vi "IDToSubnetAddress.vi"() -> ()   [LabVIEW 2016]
uses:
  ILCID.ctl
panel:
  out "Address":i16
  out "Subnet":i16
  in  "ILCID":T1
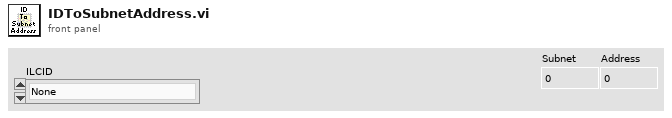
[diagram p1: front panel]
types:
  T1 = typedef "ILCID.ctl" = enum8{"None", "HP1", "HP2", "HP3", "HP4", "HP5", "HP6", "HM1", "HM2", "HM3", "HM4", "HM5", "HM6", "FA101", "FA102", "FA103", "FA104", "FA105", "FA106", "FA107", "FA108", "FA109", "FA110", "FA111", "FA112", "FA113", "FA114", "FA115", "FA116", "FA117", "FA118", "FA119", "FA120", "FA121", "FA122", "FA123", "FA124", "FA125", "FA126", "FA127", "FA128", "FA129", "FA130", "FA131", "FA132", "FA133", "FA134", "FA135", "FA136", "FA137", "FA138", "FA139", "FA140", "FA141", "FA142", "FA143", "FA207", "FA208", "FA209", "FA210", "FA211", "FA212", "FA214", "FA215", "FA216", "FA217", "FA218", "FA219", "FA220", "FA221", "FA222", "FA223", "FA224", "FA225", "FA227", "FA228", "FA229", "FA230", "FA231", "FA232", "FA233", "FA234", "FA235", "FA236", "FA237", "FA238", "FA239", "FA240", "FA241", "FA242", "FA243", "FA301", "FA302", "FA303", "FA304", "FA305", "FA306", "FA307", "FA308", "FA309", "FA310", "FA311", "FA312", "FA313", "FA314", "FA315", "FA316", "FA317", "FA318", "FA319", "FA320", "FA321", "FA322", "FA323", "FA324", "FA325", "FA326", "FA327", "FA328", "FA329", "FA330", "FA331", "FA332", "FA333", "FA334", "FA335", "FA336", "FA337", "FA338", "FA339", "FA340", "FA341", "FA342", "FA343", "FA407", "FA408", "FA409", "FA410", "FA411", "FA412", "FA414", "FA415", "FA416", "FA417", "FA418", "FA419", "FA420", "FA421", "FA422", "FA423", "FA424", "FA425", "FA427", "FA428", "FA429", "FA430", "FA431", "FA432", "FA433", "FA434", "FA435", "FA436", "FA437", "FA438", "FA439", "FA440", "FA441", "FA442", "FA443"}
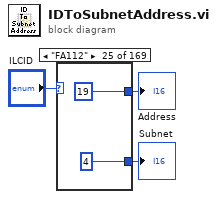
[diagram p0: block diagram]
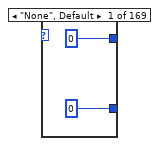
[diagram p2: hidden frame]
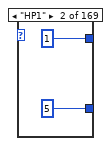
[diagram p3: hidden frame]
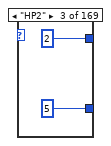
[diagram p4: hidden frame]
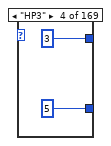
[diagram p5: hidden frame]
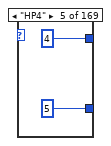
[diagram p6: hidden frame]
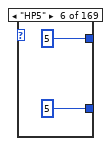
[diagram p7: hidden frame]
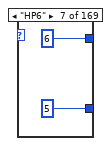
[diagram p8: hidden frame]
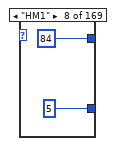
[diagram p9: hidden frame]
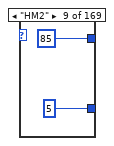
[diagram p10: hidden frame]
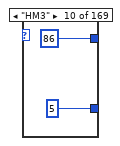
[diagram p11: hidden frame]
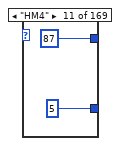
[diagram p12: hidden frame]
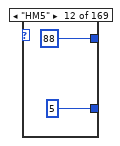
[diagram p13: hidden frame]
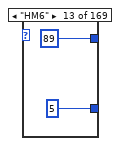
[diagram p14: hidden frame]
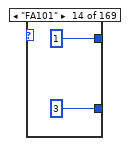
[diagram p15: hidden frame]
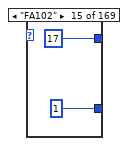
[diagram p16: hidden frame]
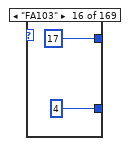
[diagram p17: hidden frame]
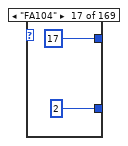
[diagram p18: hidden frame]
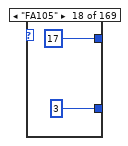
[diagram p19: hidden frame]
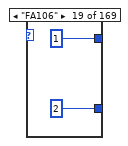
[diagram p20: hidden frame]
diagram:
  n1 = case shown="\"FA112\"" "ILCID" {
    tunnel: [i16 0 i16 5 i16 5 i16 5 i16 5 i16 5 i16 5 i16 5 i16 5 i16 5 i16 5 i16 5 i16 5 i16 3 i16 1 i16 4 i16 2 i16 3 i16 2 i16 1 i16 4 i16 2 i16 3 i16 1 i16 4 i16 2 i16 3 i16 1 i16 4 i16 2 i16 3 i16 2 i16 1 i16 4 i16 2 i16 3 i16 1 i16 4 i16 2 i16 3 i16 1 i16 4 i16 2 i16 3 i16 1 i16 4 i16 2 i16 3 i16 4 i16 2 i16 3 i16 1 i16 4 i16 1 i16 2 i16 3 i16 1 i16 4 i16 2 i16 3 i16 1 i16 4 i16 3 i16 1 i16 4 i16 2 i16 3 i16 2 i16 1 i16 4 i16 2 i16 3 i16 1 i16 4 i16 3 i16 1 i16 4 i16 2 i16 3 i16 1 i16 4 i16 2 i16 3 i16 4 i16 2 i16 3 i16 1 i16 4 i16 1 i16 2 i16 3 i16 3 i16 1 i16 4 i16 2 i16 3 i16 2 i16 1 i16 4 i16 2 i16 3 i16 1 i16 4 i16 2 i16 3 i16 1 i16 4 i16 2 i16 3 i16 2 i16 1 i16 4 i16 2 i16 3 i16 1 i16 4 i16 2 i16 3 i16 1 i16 4 i16 2 i16 3 i16 1 i16 4 i16 2 i16 3 i16 4 i16 2 i16 3 i16 1 i16 4 i16 1 i16 2 i16 3 i16 1 i16 4 i16 2 i16 3 i16 1 i16 4 i16 3 i16 1 i16 4 i16 2 i16 3 i16 2 i16 1 i16 4 i16 2 i16 3 i16 1 i16 4 i16 3 i16 1 i16 4 i16 2 i16 3 i16 1 i16 4 i16 2 i16 3 i16 4 i16 2 i16 3 i16 1 i16 4 i16 1 i16 2 i16 3] -> w2
    tunnel: [i16 0 i16 1 i16 2 i16 3 i16 4 i16 5 i16 6 i16 84 i16 85 i16 86 i16 87 i16 88 i16 89 i16 1 i16 17 i16 17 i16 17 i16 17 i16 1 i16 1 i16 18 i16 18 i16 18 i16 18 i16 19 i16 19 i16 19 i16 19 i16 19 i16 20 i16 20 i16 2 i16 20 i16 21 i16 21 i16 21 i16 21 i16 1 i16 22 i16 22 i16 22 i16 22 i16 23 i16 2 i16 23 i16 23 i16 24 i16 23 i16 2 i16 25 i16 24 i16 2 i16 3 i16 3 i16 3 i16 3 i16 4 i16 24 i16 26 i16 24 i16 24 i16 25 i16 26 i16 25 i16 26 i16 27 i16 27 i16 4 i16 26 i16 27 i16 28 i16 28 i16 27 i16 4 i16 29 i16 28 i16 28 i16 29 i16 4 i16 29 i16 29 i16 30 i16 30 i16 5 i16 31 i16 31 i16 5 i16 6 i16 6 i16 5 i16 5 i16 6 i16 30 i16 30 i16 32 i16 32 i16 6 i16 7 i16 31 i16 33 i16 33 i16 31 i16 32 i16 34 i16 34 i16 32 i16 33 i16 35 i16 35 i16 7 i16 33 i16 34 i16 36 i16 36 i16 34 i16 7 i16 37 i16 37 i16 35 i16 35 i16 38 i16 7 i16 36 i16 36 i16 39 i16 38 i16 8 i16 40 i16 39 i16 8 i16 9 i16 9 i16 8 i16 8 i16 10 i16 37 i16 41 i16 40 i16 37 i16 38 i16 41 i16 38 i16 39 i16 42 i16 42 i16 9 i16 39 i16 40 i16 43 i16 43 i16 40 i16 10 i16 44 i16 41 i16 41 i16 44 i16 9 i16 42 i16 42 i16 45 i16 45 i16 11 i16 26 i16 46 i16 11 i16 12 i16 12 i16 10 i16 10] -> w1
    frame "None", Default {
    }
    frame "HP1" {
    }
    frame "HP2" {
    }
    frame "HP3" {
    }
    frame "HP4" {
    }
    frame "HP5" {
    }
    frame "HP6" {
    }
    frame "HM1" {
    }
    frame "HM2" {
    }
    frame "HM3" {
    }
    frame "HM4" {
    }
    frame "HM5" {
    }
    frame "HM6" {
    }
    frame "FA101" {
    }
    frame "FA102" {
    }
    frame "FA103" {
    }
    frame "FA104" {
    }
    frame "FA105" {
    }
    frame "FA106" {
    }
    frame "FA107" {
    }
    frame "FA108" {
    }
    frame "FA109" {
    }
    frame "FA110" {
    }
    frame "FA111" {
    }
    frame "FA112" {
    }
    frame "FA113" {
    }
    frame "FA114" {
    }
    frame "FA115" {
    }
    frame "FA116" {
    }
    frame "FA117" {
    }
    frame "FA118" {
    }
    frame "FA119" {
    }
    frame "FA120" {
    }
    frame "FA121" {
    }
    frame "FA122" {
    }
    frame "FA123" {
    }
    frame "FA124" {
    }
    frame "FA125" {
    }
    frame "FA126" {
    }
    frame "FA127" {
    }
    frame "FA128" {
    }
    frame "FA129" {
    }
    frame "FA130" {
    }
    frame "FA131" {
    }
    frame "FA132" {
    }
    frame "FA133" {
    }
    frame "FA134" {
    }
    frame "FA135" {
    }
    frame "FA136" {
    }
    frame "FA137" {
    }
    frame "FA138" {
    }
    frame "FA139" {
    }
    frame "FA140" {
    }
    frame "FA141" {
    }
    frame "FA142" {
    }
    frame "FA143" {
    }
    frame "FA207" {
    }
    frame "FA208" {
    }
    frame "FA209" {
    }
    frame "FA210" {
    }
    frame "FA211" {
    }
    frame "FA212" {
    }
    frame "FA214" {
    }
    frame "FA215" {
    }
    frame "FA216" {
    }
    frame "FA217" {
    }
    frame "FA218" {
    }
    frame "FA219" {
    }
    frame "FA220" {
    }
    frame "FA221" {
    }
    frame "FA222" {
    }
    frame "FA223" {
    }
    frame "FA224" {
    }
    frame "FA225" {
    }
    frame "FA227" {
    }
    frame "FA228" {
    }
    frame "FA229" {
    }
    frame "FA230" {
    }
    frame "FA231" {
    }
    frame "FA232" {
    }
    frame "FA233" {
    }
    frame "FA234" {
    }
    frame "FA235" {
    }
    frame "FA236" {
    }
    frame "FA237" {
    }
    frame "FA238" {
    }
    frame "FA239" {
    }
    frame "FA240" {
    }
    frame "FA241" {
    }
    frame "FA242" {
    }
    frame "FA243" {
    }
    frame "FA301" {
    }
    frame "FA302" {
    }
    frame "FA303" {
    }
    frame "FA304" {
    }
    frame "FA305" {
    }
    frame "FA306" {
    }
    frame "FA307" {
    }
    frame "FA308" {
    }
    frame "FA309" {
    }
    frame "FA310" {
    }
    frame "FA311" {
    }
    frame "FA312" {
    }
    frame "FA313" {
    }
    frame "FA314" {
    }
    frame "FA315" {
    }
    frame "FA316" {
    }
    frame "FA317" {
    }
    frame "FA318" {
    }
    frame "FA319" {
    }
    frame "FA320" {
    }
    frame "FA321" {
    }
    frame "FA322" {
    }
    frame "FA323" {
    }
    frame "FA324" {
    }
    frame "FA325" {
    }
    frame "FA326" {
    }
    frame "FA327" {
    }
    frame "FA328" {
    }
    frame "FA329" {
    }
    frame "FA330" {
    }
    frame "FA331" {
    }
    frame "FA332" {
    }
    frame "FA333" {
    }
    frame "FA334" {
    }
    frame "FA335" {
    }
    frame "FA336" {
    }
    frame "FA337" {
    }
    frame "FA338" {
    }
    frame "FA339" {
    }
    frame "FA340" {
    }
    frame "FA341" {
    }
    frame "FA342" {
    }
    frame "FA343" {
    }
    frame "FA407" {
    }
    frame "FA408" {
    }
    frame "FA409" {
    }
    frame "FA410" {
    }
    frame "FA411" {
    }
    frame "FA412" {
    }
    frame "FA414" {
    }
    frame "FA415" {
    }
    frame "FA416" {
    }
    frame "FA417" {
    }
    frame "FA418" {
    }
    frame "FA419" {
    }
    frame "FA420" {
    }
    frame "FA421" {
    }
    frame "FA422" {
    }
    frame "FA423" {
    }
    frame "FA424" {
    }
    frame "FA425" {
    }
    frame "FA427" {
    }
    frame "FA428" {
    }
    frame "FA429" {
    }
    frame "FA430" {
    }
    frame "FA431" {
    }
    frame "FA432" {
    }
    frame "FA433" {
    }
    frame "FA434" {
    }
    frame "FA435" {
    }
    frame "FA436" {
    }
    frame "FA437" {
    }
    frame "FA438" {
    }
    frame "FA439" {
    }
    frame "FA440" {
    }
    frame "FA441" {
    }
    frame "FA442" {
    }
    frame "FA443" {
    }
  }
  "Subnet" <- w2
  "Address" <- w1
